vi "Save_to_Project.vi"(8 "error in (no error)":errorcluster, 9 "index":i32, 10 "buildObject":T1, 11 "AB_Source_ExportedVI in":refnum<class "AB_Source_ExportedVI.lvclass">) -> (0 "error out":errorcluster, 3 "AB_Source_ExportedVI out":refnum<class "AB_Source_ExportedVI.lvclass">)   [LabVIEW 2020, in "AB_Source_ExportedVI.lvclass"]
uses:
  <vilib>/AppBuilder/AB_Classes/Source/ExportedVI/AB_Source_ExportedVI.lvclass
  <resource>/Framework/Providers/API/ItemRef.ctl
  <vilib>/AppBuilder/RW_Project/AB_RW_Project_Source_ExportedVI_Data_New.ctl
  <vilib>/AppBuilder/ABAPI Dist VI Proto Info New.ctl
  <vilib>/AppBuilder/RW_Project/AB_RW_Project_PropBag_Action.ctl
  <vilib>/AppBuilder/AB_Classes/Source/ExportedVI/AB_Source_ExportedVI.lvclass/AB_Source_ExportedVI.ctl
  <vilib>/AppBuilder/AB_Classes/Source/VI/AB_Source_VI.lvclass
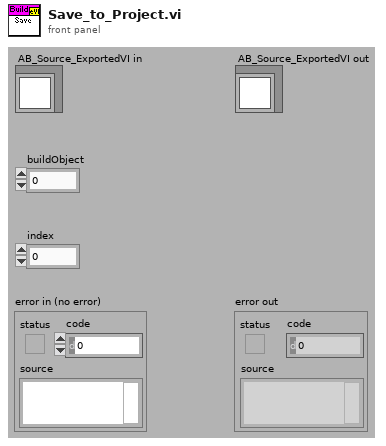
[diagram p1: front panel]
types:
  T1 = typedef "ItemRef.ctl" = u64
  T2 = typedef "AB_RW_Project_Source_ExportedVI_Data_New.ctl" = cluster{"vipInfo":T3}
  T3 = typedef "ABAPI Dist VI Proto Info New.ctl" = cluster{"cptm":string, "params":cluster{"name":string, "dir":enum32{"in", "out", "in/out", "length", "error-out"}, "inputIdx":i32, "outputIdx":i32, "passBy":i32, "lenInput":i32, "lenOutput":i32}[], "callingConv":i32, "name":string, "Description":string, "isCustomDesc":i32}
  T4 = typedef "AB_RW_Project_PropBag_Action.ctl" = enum16{"read", "write", "clear", "readPrevious", "writePrevious", "clearPrevious"}
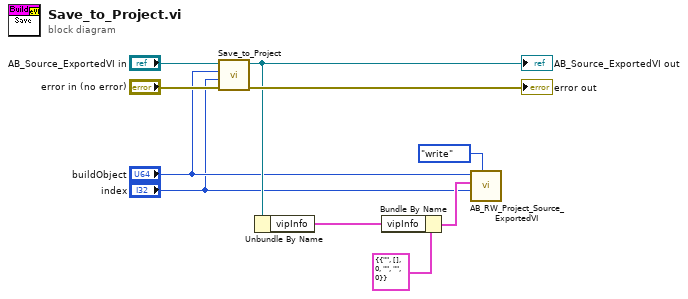
[diagram p0: block diagram]
diagram:
  n1 = call-parent "Save_to_Project.vi"("error in (no error)"="error in (no error)", "index"="index", "buildObject"="buildObject", "AB_Source_VI in"="AB_Source_ExportedVI in") -> ("error out"=→"error out":errorcluster, "AB_Source_VI out"=w6:refnum<class "AB_Source_ExportedVI.lvclass">)  [unwired: 6 in]
  "AB_Source_ExportedVI out" <- w6
  n2 = Unbundle By Name(w6) -> ("vipInfo"=w5:T3)
  n3 = Bundle By Name(cluster=T2 {"vipInfo"={"cptm"="", "params"=[], "callingConv"=0, "name"="", "Description"="", "isCustomDesc"=0}} ("dataSourceExportedVI"), "vipInfo"=w5) -> (w4:T2)
  n4 = call <vilib>:"AB_RW_Project_Source_ExportedVI.vi"("action"=AB_RW_Project_PropBag_Action."write", "index in"="index", "dataSource in"=w4, "buildObject"="buildObject") -> ()  [unwired: 4 in, 4 out]
